vi "Read Curent Temperature.vi"(11 "XML Handler in":refnum<class "XML Handler.lvclass">) -> (2 "Curent Temperature":refnum<k20>, 3 "XML Handler out":refnum<class "XML Handler.lvclass">)   [LabVIEW 2020, in "XML Handler.lvclass"]
uses:
  XML Handler.lvclass
  XML Handler.lvclass/XML Handler.ctl
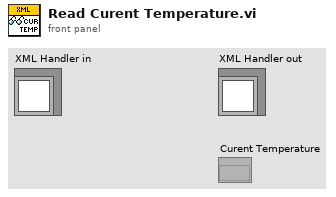
[diagram p1: front panel]
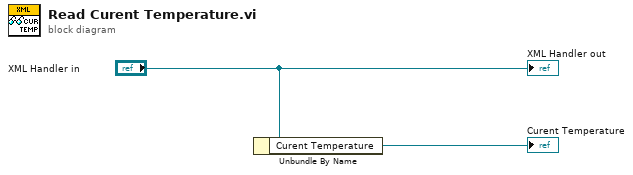
[diagram p0: block diagram]
diagram:
  n1 = Unbundle By Name("XML Handler in") -> ("Curent Temperature"=→"Curent Temperature":refnum<k20>)
  "XML Handler out" <- "XML Handler in"
